vi "Build State String with Arguments++.vi"(5 "State":string, 7 "Arguments (\"\")":string, 9 "Target Module (\"\")":string, 12 "Type":T1) -> (6 "CSM Message String":string)   [LabVIEW 2017, in "Communicable State Machine.lvlib"]
doc: "This VI is obsolete. Please use `Build Message with Arguments++.vi`\n\n## Build Message with Arguments++.vi\nBuilds CSM message strings and operation strings.\n\n> - Ref: Message Building API\n\n> [!NOTE] <b>Polymorphic VI Options</b>\n> - Build Message with Arguments(Auto Check).vi: Concatenates message strings based on the input message symbols.\n> - Build Asynchronous Message with Arguments.vi: Concatenates and generates CSM asynchronous message strings. The message type symbol is `->`.\n> - Build No-Reply Asynchronous Message with Arguments.vi: Concatenates and generates CSM asynchronous message strings without reply. The message type symbol is `->|`.\n> - Build Synchronous Message with Arguments.vi: Concatenates and generates CSM synchronous message strings. The message type symbol is `-@`.\n> - Build Interrupt Broadcast Message.vi: Concatenates and generates CSM interrupt broadcast strings.\n> - Build Normal Broadcast Message.vi: Concatenates and generates CSM status broadcast strings.\n> - Build Register Message.vi: Concatenates and generates CSM register state operation strings.\n> - Build Unregister Message.vi: Concatenates and generates CSM unregister state operation strings.\n> - CSM - Replace Marks in Messages.vi: Replaces placeholders in message strings.\n> - CSM - Replace Mark with String Array.vi: Replaces tags in a single state string with strings from an array and merges them into a string describing a group of states.\n\n> - Ref: CSM Inter-module Communication Types\n\n### Build Message with Arguments(Auto Check).vi\nConcatenates and generates CSM message strings. The message type symbol is automatically detected based on the input <b>State with Arguments</b>.\n\n> - Ref: Message Building API\n> - Ref: CSM Message Target Module Description\n\n-- <b>Controls</b> --\n- <b>State with Arguments</b>: CSM state string, which can contain arguments and target module information.\n- <b>Arguments (\"\")</b>: Argument information. Arguments contained in <b>State with Arguments</b> will be replaced.\n- <b>Target Module (\"\")</b>: Target module. If empty, the default module in <b>State with Arguments</b> will be used.\n\n-- <b>Indicators</b> --\n- <b>CSM Message String</b>: Concatenated CSM message string.\n\n### Build Synchronous Message with Arguments.vi\nConcatenates and generates CSM synchronous message strings. The message type symbol is `-@`, for example:\n\n Message >> Arguments -@ Target\n\n> - Ref: Message Building API\n> - Ref: Synchronous Message\n> - Ref: CSM Message Target Module Description\n\n-- <b>Controls</b> --\n- <b>State with Arguments</b>: CSM state string.\n- <b>Arguments (\"\")</b>: Argument information. Arguments contained in <b>State with Arguments</b> will be replaced.\n- <b>Target Module (\"\")</b>: Target module. If empty, the default module in <b>State with Arguments</b> will be used.\n\n-- <b>Indicators</b> --\n- <b>CSM Message String</b>: Concatenated CSM message string.\n\n### Build Asynchronous Message with Arguments.vi\nConcatenates and generates CSM asynchronous message strings. The message type symbol is `->`, for example:\n\n Message >> Arguments -> Target\n\n> - Ref: Message Building API\n> - Ref: Asynchronous Message\n> - Ref: CSM Message Target Module Description\n\n-- <b>Controls</b> --\n- <b>State with Arguments</b>: CSM state string.\n- <b>Arguments (\"\")</b>: Argument information. Arguments contained in <b>State with Arguments</b> will be replaced.\n- <b>Target Module (\"\")</b>: Target module. If empty, the default module in <b>State with Arguments</b> will be used.\n\n-- <b>Indicators</b> --\n- <b>CSM Message String</b>: Concatenated CSM message string.\n\n### Build No-Reply Asynchronous Message with Arguments.vi\nConcatenates and generates CSM asynchronous message strings without reply. The message type symbol is `->|`, for example:\n\n Message >> Arguments ->| Target\n\n> - Ref: Message Building API\n> - Ref: Asynchronous Message\n> - Ref: CSM Message Target Module Description\n\n-- <b>Controls</b> --\n- <b>State with Arguments</b>: CSM state string.\n- <b>Arguments (\"\")</b>: Argument information. Arguments contained in <b>State with Arguments</b> will be replaced.\n- <b>Target Module (\"\")</b>: Target module. If empty, the default module in <b>State with Arguments</b> will be used.\n\n-- <b>Indicators</b> --\n- <b>CSM Message String</b>: Concatenated CSM message string.\n\n### Build Status Broadcast Message.vi\nConcatenates normal status message strings. The message format is as follows:\n\n Status >> Arguments -><status>\n // The following strings are equivalent operations.\n // More operation characters are defined for easier typing and memorization.\n Status >> Arguments -><broadcast>\n Status >> Arguments -><all>\n\n> - Ref: Message Building API\n\n-- <b>Controls</b> --\n- <b>State with Arguments</b>: CSM normal status message string.\n- <b>Arguments (\"\")</b>: Argument information. Arguments contained in <b>State with Arguments</b> will be replaced.\n\n-- <b>Indicators</b> --\n- <b>CSM Message String</b>: Concatenated CSM message string.\n\n### Build Interrupt Broadcast Message.vi\nConcatenates interrupt status messages. The message format is as follows:\n\n Status >> Arguments -><interrupt>\n\n> - Ref: Message Building API\n\n-- <b>Controls</b> --\n- <b>State with Arguments</b>: CSM interrupt status message string.\n- <b>Arguments (\"\")</b>: Argument information. Arguments contained in <b>State with Arguments</b> will be replaced.\n\n-- <b>Indicators</b> --\n- <b>CSM Message String</b>: Concatenated CSM message string.\n\n### Build Register Message.vi\nConcatenates register state operation message strings. The message format is as follows:\n\n //[source-state]@[source-module] >> [response-message]@[response-module] -><register>\n status @ Source >> API @ Target -><register>\n\n Example: Bind the \"Download Finished\" message of the Downloader module to the \"Start Play\" API of the Player module.\n // Bind the \"Download Finished\" message of the Downloader module to the \"Start Play\" API of the Player module\n DownloadFinished@Downloader >> StartPlay@Player -><register>\n // When executing the message within the Player module, \"Player\" can be omitted\n DownloadFinished@Downloader >> StartPlay -><register>\n // When multiple modules have the \"Download Finished\" message,\n // use * to bind this message from all modules to the \"Start Play\" API of the Player module\n DownloadFinished@* >> StartPlay@Player -><register>\n\n> - Ref: Message Building API\n> - Ref: CSM Registration\n> - Ref: CSM Registration Location\n> - Ref: CSM Broadcast Priority\n\n-- <b>Controls</b> --\n- <b>Target CSM</b>: Name of the CSM module registering to the status.\n- <b>Source CSM (* as Default)</b>: Name of the CSM module publishing the status.\n- <b>Status</b>: Status to register.\n- <b>API (If \"\", Same As \"Status\")</b>: Name of the API in the registering module that responds to the status.\n- <b>Priority (No Change)</b>: Priority of the broadcast after registration.\n\n-- <b>Indicators</b> --\n- <b>CSM Message String</b>: Concatenated CSM message string.\n\n### Build Unregister Message.vi\nConcatenates unregister state operation message strings. The message format is as follows:\n\n //[source-state]@[source-module] >> [response-message]@[response-module] -><unregister>\n status @ Source >> API @ Target -><unregister>\n\n Example: Cancel the binding of the \"Download Finished\" message of the Downloader module to the \"Start Play\" API of the Player module.\n // Cancel binding of the \"Download Finished\" message of the Downloader module to the \"Start Play\" API of the Player module\n DownloadFinished@Downloader >> StartPlay@Player -><unregister>\n // When executing the message within the Player module, \"Player\" can be omitted\n DownloadFinished@Downloader >> StartPlay -><unregister>\n\n- In Worker Mode, the module's internal registration rules will only be automatically unregistered after all nodes have exited.\n- In Chain of Responsibility Mode, the module's internal registration rules will be automatically unregistered as the node exits.\n\n> - Ref: Message Building API\n> - Ref: CSM Registration\n> - Ref: CSM Registration Location\n\n-- <b>Controls</b> --\n- <b>Target CSM</b>: Name of the CSM module registering to the status.\n- <b>Source CSM (* as Default)</b>: Name of the CSM module publishing the status.\n- <b>Status</b>: Registered status.\n- <b>API (If \"\", Same As \"Status\")</b>: Name of the API in the registering module that responds to the status to be unregistered.\n\n-- <b>Indicators</b> --\n- <b>CSM Message String</b>: Concatenated CSM message string.\n\n### CSM - Replace Marks in Messages.vi\nFacilitates editing multiple CSM message strings by providing a batch replacement function for marks. There are four marks that can be replaced:\n- `<param>` mark: Usually represents the same argument.\n- `<target>` mark: Usually represents the same target.\n- `<1>` mark: Represents custom mark 1.\n- `<2>` mark: Represents custom mark 2.\n\n<b>Example</b>: The terminal `<target>` is connected to the string `DAQDevice`. The <b>States with Replace Token</b> string is:\n\n text\n Initialize -@ <target>\n Configure -@ <target>\n Read -@ <target>\n Close -@ <target>\n\nThe <b>States</b> output is:\n\n text\n Initialize -@ DAQDevice\n Configure -@ DAQDevice\n Read -@ DAQDevice\n Close -@ DAQDevice\n\n> - Ref: Message Building API\n\n-- <b>Controls</b> --\n- <b>States with Replace Token</b>: CSM state string with replacement marks.\n- <b><param></b>: `<param>` mark, which usually represents the same argument.\n- <b><target></b>: `<target>` mark, which usually represents the same target.\n- <b><1></b>: Custom mark 1.\n- <b><2></b>: Custom mark 2.\n\n-- <b>Indicators</b> --\n- <b>States</b>: State string after replacement.\n\n### CSM - Replace Mark with String Array.vi\nReplaces tags in a single state string with strings from an array and merges them into a string describing a group of states.\n\n<b>Example</b>: For `Draw >> <1> -@ Painter`, <b>Tag</b> should be set to `<1>`\n\nInput array `[Line, Circle, Rectangle]`. The result will be:\n\n Draw >> Line -@ Painter\n Draw >> Circle -@ Painter\n Draw >> Rectangle -@ Painter\n\n-- <b>Controls</b> --\n- <b>single-line text</b>: Single-line state string containing tags like `<1>`, `<2>`, `<3>`, etc.\n- <b>Substitution Mark</b>: The tag to replace, such as `<1>`, `<2>`, `<3>`, etc.\n- <b>replace string</b>: The array of strings to replace the tag with.\n\n-- <b>Indicators</b> --\n- <b>States</b>: The merged state string."
uses:
  Communicable State Machine.lvlib
  AdvanceAPI/CSM - Message Type.ctl
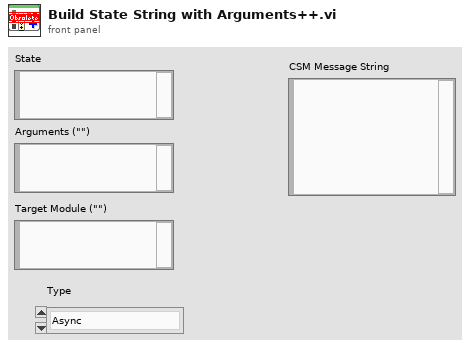
[diagram p1: front panel]
types:
  T1 = typedef "Communicable State Machine.lvlib/CSM - Message Type.ctl" = enum16{"Async", "Async without Reply", "Sync"}
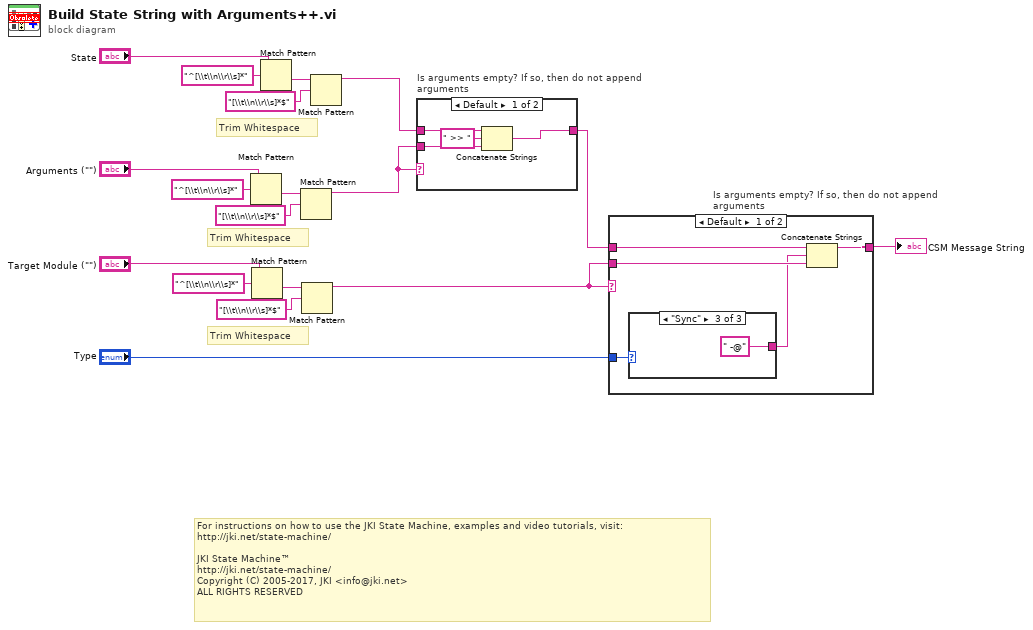
[diagram p0: block diagram]
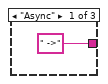
[diagram p2: hidden frame]
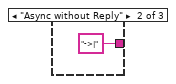
[diagram p3: hidden frame]
diagram:
  # "Trim Whitespace"
  # "Trim Whitespace"
  # "For instructions on how to use the JKI State Machine, examples and video tutorials, visit:\nhttp://jki.net/state-machine/\n\nJKI State Machine™\nhttp://jki.net/state-machine/\nCopyright (C) 2005-2017, JKI <info@jki.net>\nALL RIGHTS RESERVED"
  # "Trim Whitespace"
  n1 = Match Pattern(string="Arguments (\"\")", regular expression="^[\\t\\n\\r\\s]*") -> (after substring=w12:string)  [unwired: 1 in, 3 out]
  n2 = Match Pattern(string="Target Module (\"\")", regular expression="^[\\t\\n\\r\\s]*") -> (after substring=w7:string)  [unwired: 1 in, 3 out]
  n3 = Match Pattern(string="State", regular expression="^[\\t\\n\\r\\s]*") -> (after substring=w17:string)  [unwired: 1 in, 3 out]
  n4 = Match Pattern(string=w12, regular expression="[\\t\\n\\r\\s]*$") -> (before substring=w9:string)  [unwired: 1 in, 3 out]
  n5 = Match Pattern(string=w7, regular expression="[\\t\\n\\r\\s]*$") -> (before substring=w4:string)  [unwired: 1 in, 3 out]
  n6 = Match Pattern(string=w17, regular expression="[\\t\\n\\r\\s]*$") -> (before substring=w14:string)  [unwired: 1 in, 3 out]
  n7 = case "Is arguments empty? If so, then do not append arguments" shown="Default" w9 {
    tunnel: [w19 w23] -> w2
    tunnel: w14 -> [w22 w23]
    tunnel: w9 -> [w20 _]
    frame Default {
      n8 = Concatenate Strings(w22, " >> " ("string"), w20) -> (w19:string)
    }
    frame "" {
    }
  }
  n9 = case "Is arguments empty? If so, then do not append arguments" shown="Default" w4 {
    tunnel: [w26 w32] -> w3
    tunnel: w2 -> [w28 w32]
    tunnel: w4 -> [w27 _]
    tunnel: "Type" -> [w25 _]
    frame Default {
      n10 = case shown="\"Sync\"" w25 {
        tunnel: [" ->" ("string") "->|" ("string") " -@" ("string")] -> w24
        frame "Async" {
        }
        frame "Async without Reply" {
        }
        frame "Sync" {
        }
      }
      n11 = Concatenate Strings(w28, w24, w27) -> (w26:string)
    }
    frame "" {
    }
  }
  "CSM Message String" <- w3
